vi "Property Node (XNET UDP Socket).vi"   [LabVIEW 2018]
doc: "Provides properties that can be used with the XNET UDP Socket VIs."
uses:
  <resource>/objmgr/xnet.rc
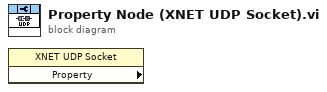
[diagram p0: block diagram]
diagram:
  n1 = property class="XNET UDP Socket" props=[]() -> ()  [unwired: 2 in, 3 out]
